vi "UnLoad.vi"(8 "error in (no error)":errorcluster) -> (0 "error out":errorcluster)   [LabVIEW 2017, in "WebServiceImporter.lvlib" / "Main Panel.lvlib" / "Finish.lvlib"]
uses:
  <vilib>/Platform/WebService/Main Panel/Pages/Finish/Finish.lvlib
  <vilib>/Platform/WebService/Main Panel/Pages/Finish/Events/Events.lvlib
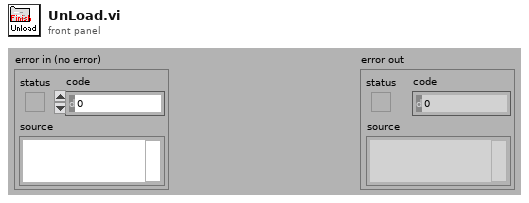
[diagram p1: front panel]
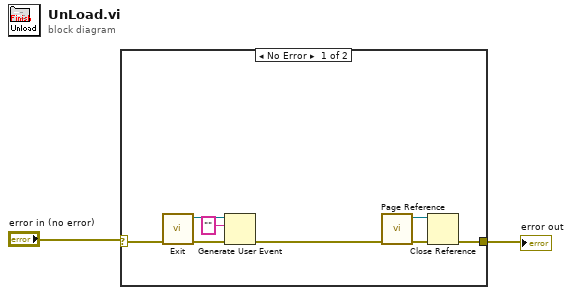
[diagram p0: block diagram]
diagram:
  n1 = case shown="No Error" "error in (no error)" {
    selector: "error in (no error)" -> [w7 w11]
    tunnel: [w10 w11] -> w1
    frame No Error {
      n2 = call <vilib>:"Exit.vi"("error in (no error)"=w7) -> ("error out"=w5:errorcluster, "user event (out)"=w6:refnum<user-event>)  [unwired: 9 in]
      n3 = Generate User Event(user event=w6, event data cluster="" ("event data"), error in=w5) -> (error out=w3:errorcluster)  [unwired: 1 in, 1 out]
      n4 = call <vilib>:"Page Reference.vi"("error in (no error)"=w3) -> ("error out"=w8:errorcluster, "VI Refnum (out)"=w9:refnum<vi>)  [unwired: 9 in]
      n5 = Close Reference(reference=w9, error in (no error)=w8) -> (error out=w10:errorcluster)
    }
    frame Error {
    }
  }
  "error out" <- w1
